vi "WirebirdLabs-VIServer-LinkerInfo.vi"(8 "error in":errorcluster, 10 "Recursive":bool, 11 "LabVIEW Filetype":path) -> (0 "error out":errorcluster, 3 "LinkerInfo":T1[](array[typedef]) {"iState" format="%08x"; "iStyle" format="%08x"; "wStyle" format="%08x"; "buttons" format="%08x"; "viflags" format="%08x"; "viflags2" format="%08x"})   [LabVIEW 2012]
uses:
  WirebirdLabs-VIServer-LinkerInfoStructure.ctl
panel:
  # "Inputs"
  # "Outputs"
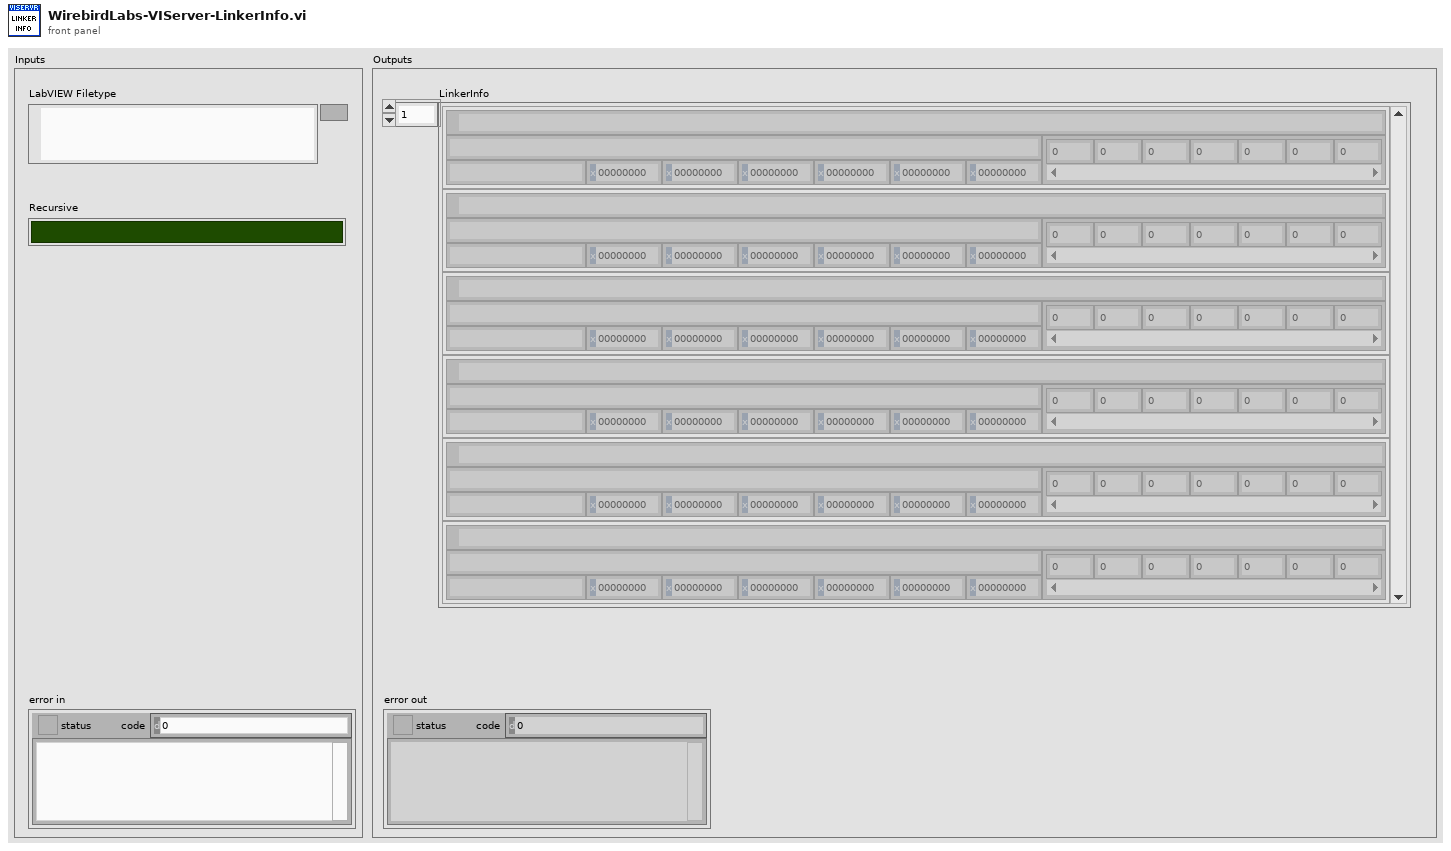
[diagram p1: front panel]
types:
  T1 = typedef "WirebirdLabs-VIServer-LinkerInfoStructure.ctl" = cluster{"path":path, "delimited name":string, "Filetype":string, "iState":u32, "iStyle":u16, "wStyle":u16, "buttons":u16, "viflags":u32, "viflags2":u32, "links":u32[]}
  T2 = typedef "NI_FileType.lvlib/LVFileType.ctl" = enum32{"Invalid file", "Unknown type", "Instrument", "Control", "Polymorphic VI", "Project", "Library", "LVClass", "XControl", "XNode", "Shared library", ".NET assembly", "ActiveX interface", "CIN", "Run-time menu", "Palette menu", "Help file", "LLB", "XNode Edit Dependency", "Class Private Data Control", "Statechart", "MathScript .m file", "Ladder Diagram", "LVLibp"}
  T3 = cluster{"path":path, "delimited name":string, "type":T2, "iState":u32, "iStyle":u16, "wStyle":u16, "buttons":u16, "viflags":u32, "viflags2":u32, "links":u32[]}[]
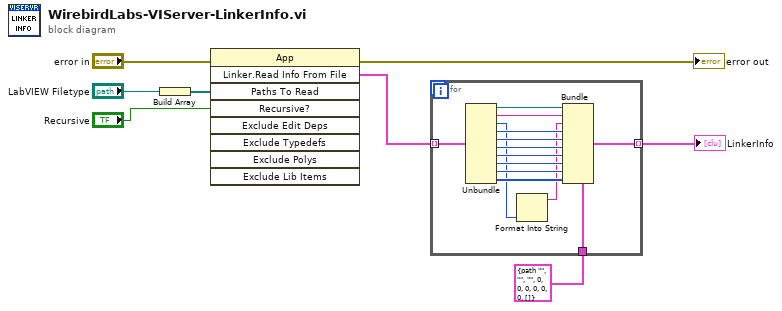
[diagram p0: block diagram]
diagram:
  n1 = Build Array("LabVIEW Filetype") -> (w7:path[])
  n2 = invoke class="App" method="Linker.Read Info From File"(error in="error in", "Paths To Read"=w7, "Recursive?"="Recursive") -> (error out=→"error out":errorcluster, "Linker.Read Info From File"=w3:T3)  [unwired: 6 in, 7 out]
  n3 = for {
    tunnel: w3 -> [w22] mode=indexing
    tunnel: [w20] -> w2 mode=indexing
    tunnel: T1 {"path"=path "", "delimited name"="", "Filetype"="", "iState"=0, "iStyle"=0, "wStyle"=0, "buttons"=0, "viflags"=0, "viflags2"=0, "links"=[]} ("Linker Info") -> [w21]
    n4 = Unbundle(w22) -> ("path"=w19:path, "delimited name"=w18:string, "type"=w10:T2, "iState"=w17:u32, "iStyle"=w16:u16, "wStyle"=w15:u16, "buttons"=w14:u16, "viflags"=w13:u32, "viflags2"=w12:u32, "links"=w11:u32[])
    n5 = Format Into String(w10) -> (resulting string=w9:string)  [unwired: 3 in, 1 out]
    n6 = Bundle(cluster=w21, "path"=w19, "delimited name"=w18, "Filetype"=w9, "iState"=w17, "iStyle"=w16, "wStyle"=w15, "buttons"=w14, "viflags"=w13, "viflags2"=w12, "links"=w11) -> (w20:T1)
  }
  "LinkerInfo" <- w2
